vi "Configure.vi"(8 "error in (no error)":errorcluster, 11 "Axsun_1310_SS in":refnum<class "Axsun_1310_SS.lvclass">) -> (0 "error out":errorcluster, 3 "Axsun_1310_SS out":refnum<class "Axsun_1310_SS.lvclass">)   [LabVIEW 2015, in "Axsun_1310_SS.lvclass"]
uses:
  Axsun_1310_SS.lvclass
  Axsun VDL Global.vi
  Laser.lvclass
types:
  T1 = enum32{"Invalid", "Standard", "Closed", "Hidden", "Minimized", "Maximized"}
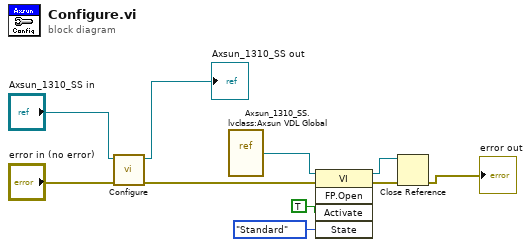
[diagram p0: block diagram]
diagram:
  n1 = call-parent "Configure.vi"("error in (no error)"="error in (no error)", "Laser in"="Axsun_1310_SS in") -> ("error out"=w4:errorcluster, "Laser out"=→"Axsun_1310_SS out":refnum<class "Axsun_1310_SS.lvclass">)  [unwired: 8 in]
  n2 = vi-ref "Axsun_1310_SS.lvclass:Axsun VDL Global.vi"() -> (w5:refnum<vi>)
  n3 = invoke class="VI" method="FP.Open"(reference=w5, error in=w4, "Activate"=TRUE ("Activate?"), "State"=T1."Standard") -> (reference out=w2:refnum<vi>, error out=w3:errorcluster)  [unwired: 1 in, 3 out]
  n4 = Close Reference(reference=w2, error in (no error)=w3) -> (error out=→"error out":errorcluster)
